vi "自加器.vi"() -> (2 "output":dbl)   [LabVIEW 2023]
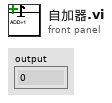
[diagram p1: front panel]
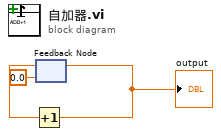
[diagram p0: block diagram]
diagram:
  n1 = feedback #1(0.0) -> (w3:dbl)
  n2 = Increment(x=w3) -> (x+1=w1:dbl)
  "output" <- w1
  n3 = feedback-in #1(w1) -> ()
